vi "拉取压缩文件并解压缩.vi"(8 "error in (no error)":errorcluster, 11 "远端地址":string="/UP/OneStation/V4/一体化微型水质监测站.zip") -> (0 "error out":errorcluster, 3 "文件路径":path)   [LabVIEW 2016, in "数据传输系统-05.lvlib" / "update.lvlib"]
uses:
  update.lvlib
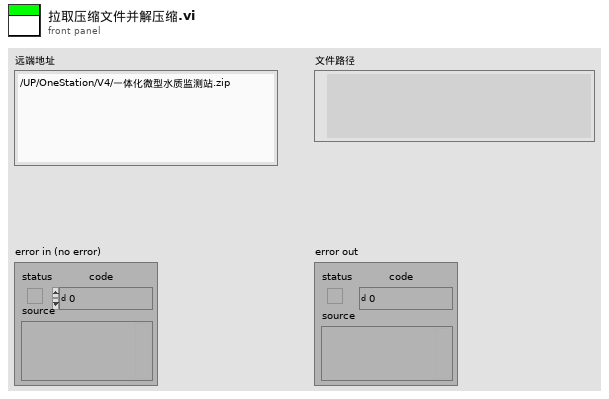
[diagram p1: front panel]
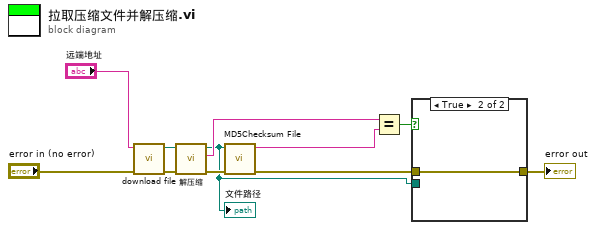
[diagram p0: block diagram]
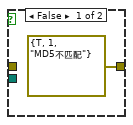
[diagram p2: hidden frame]
diagram:
  n1 = call "download file.vi"("error in (no error)"="error in (no error)", "远端地址"="远端地址") -> ("error out"=w9:errorcluster, "local file path"=w10:path)  [unwired: 8 in]
  n2 = call "解压缩.vi"("error in (no error)"=w9, "Zip file"=w10) -> ("error out"=w8:errorcluster, "MD5"=w3:string, "待校验的文件路径"=w1:path)  [unwired: 7 in]
  "文件路径" <- w1
  n3 = call <vilib>:"MD5Checksum File.vi"("error in (no error)"=w8, "Path"=w1) -> ("error out"=w6:errorcluster, "MD5 message-digest"=w2:string)  [unwired: 8 in]
  n4 = Equal?(x=w3, y=w2) -> (x = y?=w7:bool)
  n5 = case shown="True" w7 {
    tunnel: w1 -> [_ _]
    tunnel: w6 -> [_ w13]
    tunnel: [errorcluster {"status"=TRUE, "code"=1, "source"="MD5不匹配"} ("error out") w13] -> w4
    frame False {
    }
    frame True {
    }
  }
  "error out" <- w4
